vi "Set Arm.vi"(10 "Intake":enum16{"Front", "Rear"}(ring), 11 "Position":dbl format="%#_13g") -> ()   [LabVIEW 2015]
uses:
  Typedef/IntakeControllerMsg.ctl
  Typedef/IntakeControllerActions.ctl
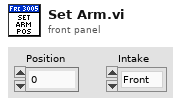
[diagram p1: front panel]
types:
  T1 = typedef "IntakeControllerActions.ctl" = enum16{"Wait on Intake Rear", "Wait on Angle Rear", "Go To Angle Rear", "Wait on Intake Front", "Wait on Angle Front", "Set Roller Front", "Set Roller Rear", "Go To Angle Front", "Wait ms"}
  T2 = typedef "IntakeControllerMsg.ctl" = cluster{"Cmd":T1, "Data":variant}
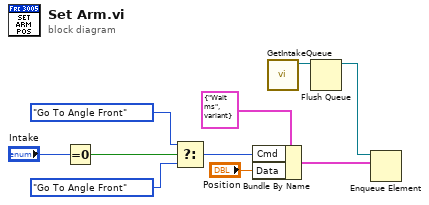
[diagram p0: block diagram]
diagram:
  n1 = Equal To 0?(x="Intake") -> (x = 0?=w5:bool)
  n2 = Select(t=IntakeControllerActions."Go To Angle Front" ("Cmd"), s=w5, f=IntakeControllerActions."Go To Angle Front" ("Cmd")) -> (s? t:f=w2:T1)
  n3 = Bundle By Name(cluster=T2 {"Cmd"=enum."Wait ms", "Data"=variant(i32 50)} ("output cluster"), "Cmd"=w2, "Data"="Position") -> (w10:T2)
  n4 = call "GetIntakeQueue.vi"() -> ("queue out"=w7:refnum<queue>)  [unwired: 11 in]
  n5 = Flush Queue(queue=w7) -> (queue out=w1:refnum<queue>)  [unwired: 1 in, 2 out]
  n6 = Enqueue Element(queue=w1, element=w10) -> ()  [unwired: 2 in, 3 out]
